vi "GNSS1-SET-4.vi"(6 "DigNum引用句柄":refnum<vi>, 9 "Ring引用句柄":refnum<vi>, 10 "Enum引用句柄":refnum<vi>, 11 "Cluster输入":refnum<vi>) -> (3 "添加的数组4":u8[](array[numeric]))   [LabVIEW 2012]
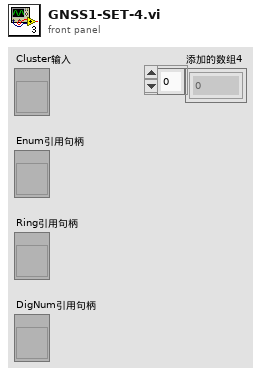
[diagram p1: front panel]
types:
  T1 = cluster{"电台通讯状态有效性":bool, "秒脉冲有效性":bool, "EFMC接收监控回绕监控字有效性":bool, "数传到接收机传输通道有效性":bool, "SPARE1":bool, "SPARE2":bool, "SPARE3":bool, "SPARE4":bool}
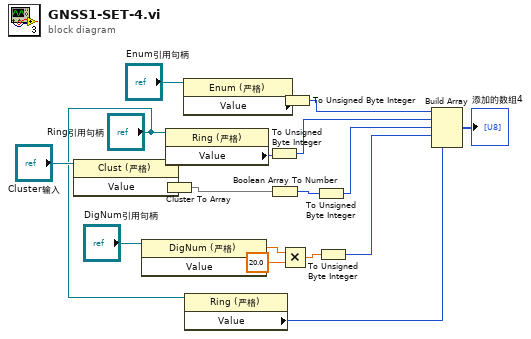
[diagram p0: block diagram]
diagram:
  n1 = property on="属性节点" class="Clust (严格)"(reference="Cluster输入") -> ("Value"=w11:T1)  [unwired: 1 in, 2 out]
  n2 = property on="属性节点" class="DigNum (严格)"(reference="DigNum引用句柄") -> ("Value"=w15:sgl)  [unwired: 1 in, 2 out]
  n3 = Cluster To Array(cluster=w11) -> (array=w9:bool[])
  n4 = property on="属性节点" class="Ring (严格)"(reference="Ring引用句柄") -> ("Value"=w5:u8)  [unwired: 1 in, 2 out]
  n5 = property on="属性节点" class="Enum (严格)"(reference="Enum引用句柄") -> ("Value"=w7:enum8{"GPS", "BD", "GLO"})  [unwired: 1 in, 2 out]
  n6 = property on="属性节点" class="Ring (严格)"(reference="Ring引用句柄") -> ("Value"=w17:u8)  [unwired: 1 in, 2 out]
  n7 = To Unsigned Byte Integer(number=w5) -> (unsigned 8bit integer=w6:u8)
  n8 = Boolean Array To Number(Boolean array=w9) -> (number=w10:u32)
  n9 = Multiply(x=w15, y=sgl 20.0) -> (x*y=w14:sgl)
  n10 = To Unsigned Byte Integer(number=w7) -> (unsigned 8bit integer=w8:u8)
  n11 = To Unsigned Byte Integer(number=w10) -> (unsigned 8bit integer=w12:u8)
  n12 = To Unsigned Byte Integer(number=w14) -> (unsigned 8bit integer=w16:u8)
  n13 = Build Array(w8, w6, w12, w16, w17) -> (→"添加的数组4":u8[])
